vi "Configure Library Classes in Memory for Development.vi"(5 "class names":string[](array[string])=["Status.lvclass", "Timing Status.lvclass", "Framework Status.lvclass", "Dispatcher Interface.lvclass", "Interface.lvclass", "Logging Interface.lvclass", "Plugin Interface.lvclass", "Error Pointer.lvclass", "ID Pool.lvclass", "Plugin Interface Pool.lvclass", "Pool.lvclass", "State.lvclass", "Data Server Thread.lvclass", "Dispatcher Thread.lvclass", "Logging Thread.lvclass", "Timing.lvclass", "Buffer Converter.lvclass", "Transceiver.lvclass", "Plugin Thread.lvclass", "Thread.lvclass", "Transceiver Thread.lvclass", "Buffer.lvclass", "Buffers.lvclass", "Performance.lvclass", "Transfer Group.lvclass", "Transfer.lvclass"], 7 "target name (My Computer)":string="My Computer", 9 "VI Options":T1={"Inline"=FALSE, "Is Reentrant"=TRUE, "Reentrancy Type"=enum."Share clones between instances", "Enable Debugging"=TRUE}, 10 "save VIs? (T)":bool=TRUE, 11 "library name":string="DSF Core.lvlib") -> (0 "error out":errorcluster)   [LabVIEW 2017, in "Build Automation.lvlib"]
uses:
  Build Automation.lvlib
  VI Options.ctl
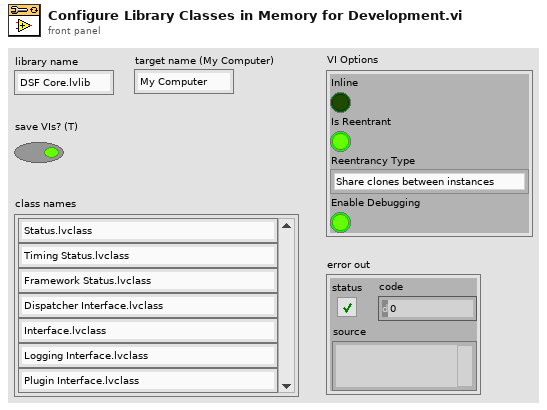
[diagram p1: front panel]
types:
  T1 = typedef "Build Automation.lvlib/VI Options.ctl" = cluster{"Inline":bool, "Is Reentrant":bool, "Reentrancy Type":enum16{"Share clones between instances", "Preallocate clone for each instance"}, "Enable Debugging":bool}
  T2 = cluster{"Status Message":refnum<data-value>, "Progress":refnum<data-value>, "Stop":refnum<data-value>}
  T3 = enum16{"Share clones between instances", "Preallocate clone for each instance"}
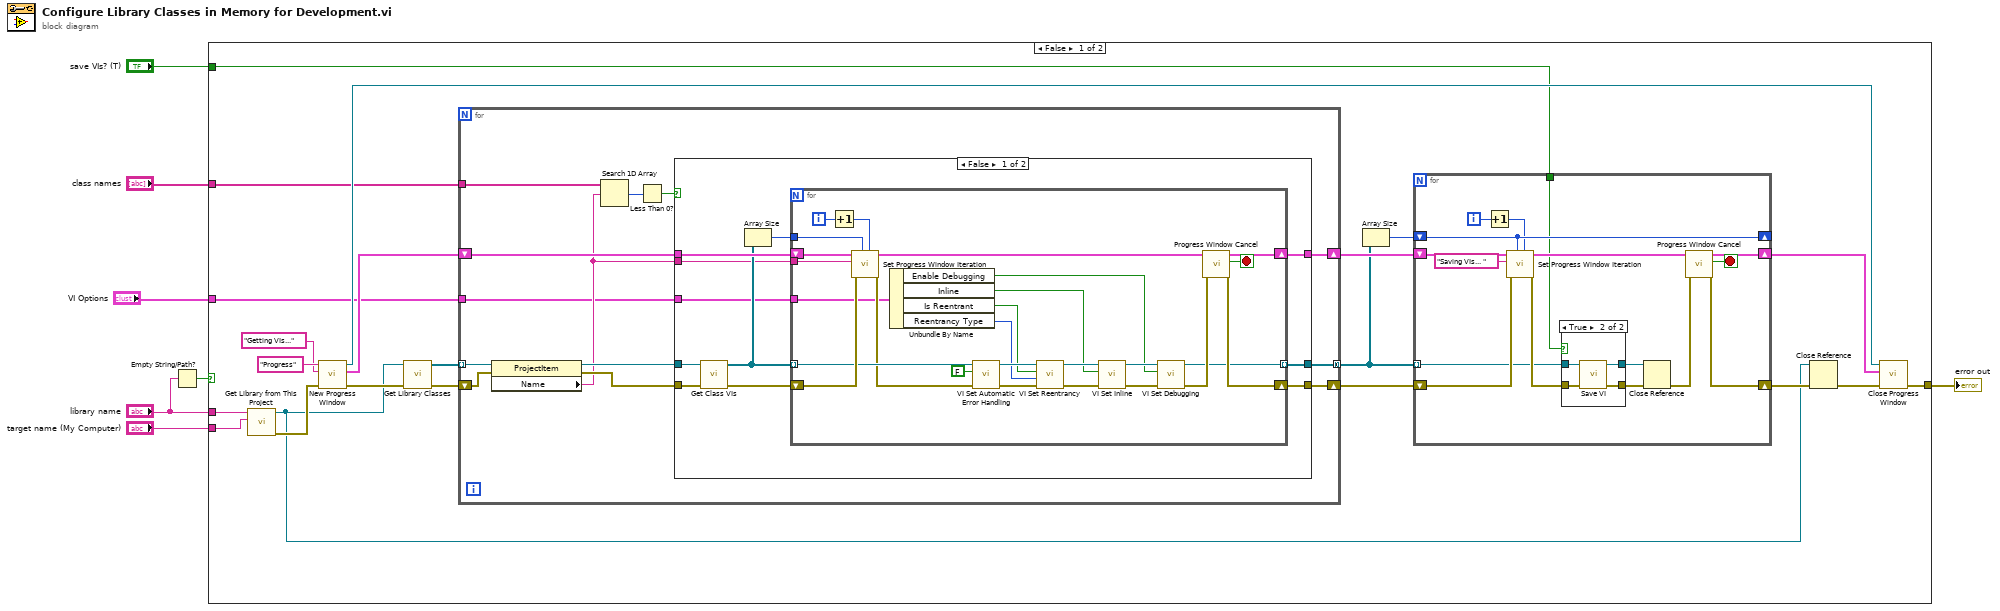
[diagram p0: block diagram]
diagram:
  n1 = Empty String/Path?(string/path="library name") -> (empty?=w7:bool)
  n2 = case shown="False" w7 {
    tunnel: [w27 _] -> w5
    tunnel: "library name" -> [w20 _]
    tunnel: "save VIs? (T)" -> [w17 _]
    tunnel: "target name (My Computer)" -> [w18 _]
    tunnel: "class names" -> [w11 _]
    tunnel: "VI Options" -> [w8 _]
    frame False {
      n3 = call "Get Library from This Project.vi"("Target Name (My Computer)"=w18, "Library Name"=w20) -> ("error out"=w19:errorcluster, "Library Refnum"=w14:refnum<vi>)  [unwired: 8 in]
      n4 = call "New Progress Window.vi"("error in (no error)"=w19, "Initial Message"="Getting VIs...", "Window Title"="Progress" ("WindowTitle")) -> ("error out"=w15:errorcluster, "DVRs"=w28:T2, "VI refnum"=w29:refnum<vi>)  [unwired: 6 in]
      n5 = call "Get Library Classes.vi"("error in (no error)"=w15, "library ref"=w14) -> ("error out"=w13:errorcluster, "class refs"=w12:refnum<vi>[])  [unwired: 7 in, 1 out]
      n6 = for {
        tunnel: [w40] -> w10 mode=concatenating
        tunnel: w12 -> [w38] mode=indexing
        shift-right: [w39] -> w25
        shift-left: w13 -> [w36]
        shift-right: [w41] -> w26
        shift-left: w28 -> [w42]
        tunnel: w11 -> [w34]
        tunnel: w8 -> [w30]
        n7 = property class="ProjectItem"(reference=w38, error in=w36) -> (reference out=w37:refnum<vi>, error out=w35:errorcluster, "Name"=w33:string)
        n8 = Search 1D Array(1D array=w34, element=w33) -> (index of element=w32:i32)  [unwired: 1 in]
        n9 = Less Than 0?(x=w32) -> (x < 0?=w31:bool)
        n10 = case shown="False" w31 {
          tunnel: w42 -> [w53 w80]
          tunnel: [w52 w80] -> w41
          tunnel: [w51 _] -> w40
          tunnel: [w50 w81] -> w39
          tunnel: w37 -> [w48 _]
          tunnel: w35 -> [w47 w81]
          tunnel: w33 -> [w45 _]
          tunnel: w30 -> [w43 _]
          frame False {
            n11 = call "Get Class VIs.vi"("error in (no error)"=w47, "class ref"=w48) -> ("error out"=w49:errorcluster, "vi refs"=w46:refnum<vi>[])  [unwired: 8 in]
            n12 = Array Size(array=w46) -> (size(s)=w44:i32)
            n13 = for {
              tunnel: w46 -> [w70] mode=indexing
              shift-right: [w77] -> w52
              shift-left: w53 -> [w74]
              shift-right: [w71] -> w50
              shift-left: w49 -> [w72]
              tunnel: [w63] -> w51 mode=indexing
              tunnel: w45 -> [w61]
              tunnel: w44 -> [w59]
              tunnel: w43 -> [w58]
              i -> [w79]
              stop <- w78 stop-if-true
              n14 = Increment(x=w79) -> (x+1=w69:i32)
              n15 = call "Set Progress Window Iteration.vi"("current iteration"=w69, "total iterations"=w59, "error in (no error)"=w72, "Status Message"=w61, "DVRs in"=w74) -> ("error out"=w60:errorcluster, "DVRs out"=w73:T2)  [unwired: 5 in]
              n16 = Unbundle By Name(w58) -> ("Enable Debugging"=w54:bool, "Inline"=w55:bool, "Is Reentrant"=w56:bool, "Reentrancy Type"=w57:T3)
              n17 = call "VI Set Automatic Error Handling.vi"("error in (no error)"=w60, "Automatic Error Handling"=FALSE, "vi ref in"=w70) -> ("error out"=w62:errorcluster, "vi ref out"=w75:refnum<vi>)  [unwired: 7 in]
              n18 = call "VI Set Reentrancy.vi"("error in (no error)"=w62, "Reentrancy Type (shared clone)"=w57, "Is Reentrant"=w56, "vi ref in"=w75) -> ("error out"=w67:errorcluster, "vi ref out"=w68:refnum<vi>)  [unwired: 6 in]
              n19 = call "VI Set Inline.vi"("error in (no error)"=w67, "Inline VI"=w55, "vi ref in"=w68) -> ("error out"=w65:errorcluster, "vi ref out"=w66:refnum<vi>)  [unwired: 7 in]
              n20 = call "VI Set Debugging.vi"("error in (no error)"=w65, "Allow Debugging"=w54, "vi ref in"=w66) -> ("error out"=w64:errorcluster, "vi ref out"=w63:refnum<vi>)  [unwired: 7 in]
              n21 = call "Progress Window Cancel.vi"("error in (no error)"=w64, "DVRs in"=w73) -> ("error out"=w71:errorcluster, "cancelled"=w78:bool, "DVRs out"=w77:T2)  [unwired: 7 in]
            }
          }
          frame True {
          }
        }
      }
      n22 = Array Size(array=w10) -> (size(s)=w9:i32)
      n23 = for {
        tunnel: w10 -> [w83] mode=indexing
        shift-right: [w95] -> w24
        shift-left: w26 -> [w94]
        shift-right: [w91] -> w22
        shift-left: w25 -> [w92]
        shift-right: [w90] -> _
        shift-left: w9 -> [w90]
        tunnel: w17 -> [w82]
        i -> [w97]
        stop <- w96 stop-if-true
        n24 = Increment(x=w97) -> (x+1=w89:i32)
        n25 = call "Set Progress Window Iteration.vi"("current iteration"=w89, "total iterations"=w90, "error in (no error)"=w92, "Status Message"="Saving VIs... ", "DVRs in"=w94) -> ("error out"=w87:errorcluster, "DVRs out"=w93:T2)  [unwired: 5 in]
        n26 = case shown="True" w82 {
          tunnel: w87 -> [w98 w103]
          tunnel: [w99 w102] -> w86
          tunnel: [w98 w101] -> w85
          tunnel: w83 -> [w99 w100]
          frame False {
          }
          frame True {
            n27 = call "Save VI.vi"("error in (no error)"=w103, "vi ref in"=w100) -> ("error out"=w101:errorcluster, "vi ref out"=w102:refnum<vi>)  [unwired: 8 in]
          }
        }
        n28 = Close Reference(reference=w86, error in (no error)=w85) -> (error out=w84:errorcluster)
        n29 = call "Progress Window Cancel.vi"("error in (no error)"=w84, "DVRs in"=w93) -> ("error out"=w91:errorcluster, "cancelled"=w96:bool, "DVRs out"=w95:T2)  [unwired: 7 in]
      }
      n30 = Close Reference(reference=w14, error in (no error)=w22) -> (error out=w21:errorcluster)
      n31 = call "Close Progress Window.vi"("error in (no error)"=w21, "DVRs in"=w24, "VI refnum"=w29) -> ("error out"=w27:errorcluster)  [unwired: 8 in]
    }
    frame True {
    }
  }
  "error out" <- w5
